vi "New Image (ARGB).vi"(7 "Colour (Default: Black)":T1={"Alpha"=255, "RGB"=0}, 8 "error in (no error)":errorcluster, 11 "Preallocated Image Size (Default: 0,0)":T3) -> (0 "error out":errorcluster, 3 "New ARGB Image":T2)   [LabVIEW 2020, in "g_ar_toolkit.image.lvlib"]
uses:
  g_ar_toolkit.image.lvlib
  g_ar_toolkit.common/Image Size (Integer).ctl
  ARGB Image.ctl
  ARGB Colour.ctl
  3321fa97-f432-4e1e-8db9-a0df79aed21b.vi
  g_ar_toolkit.common/Module Path.vi
  <vilib>/Utility/error.llb/Error Cluster From Error Code.vi
  g_ar_toolkit.common/g_ar_toolkit.common.lvlib
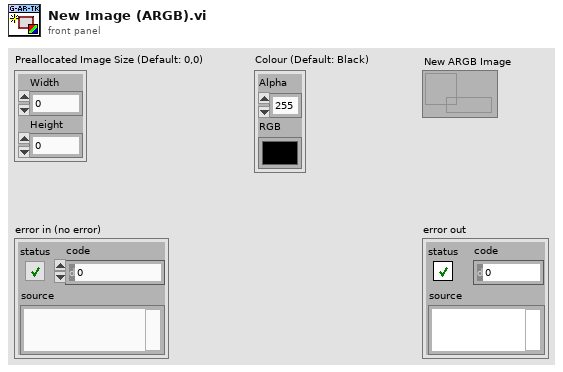
[diagram p1: front panel]
types:
  T1 = typedef "g_ar_toolkit.image.lvlib/ARGB Colour.ctl" = cluster{"Alpha":u8, "RGB":u32}
  T2 = typedef "g_ar_toolkit.image.lvlib/ARGB Image.ctl" = refnum<data-value>
  T3 = typedef "g_ar_toolkit.common.lvlib/Image Size (Integer).ctl" = cluster{"Width":u16, "Height":u16}
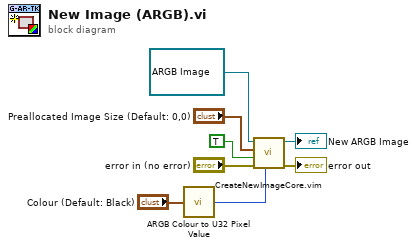
[diagram p0: block diagram]
diagram:
  n1 = call "ARGB Colour to U32 Pixel Value.vi"("ARGB Colour"="Colour (Default: Black)") -> ("U32 Colour"=w1:u32)
  n2 = call "CreateNewImageCore.vim"("Initial Value"=w1, "error in (no error)"="error in (no error)", "Is ARGB"=TRUE, "Preallocated Image Size"="Preallocated Image Size (Default: 0,0)", "Ref Type"=T2 refnum ("EDVR")) -> ("error out"=→"error out":errorcluster, "New Reference"=→"New ARGB Image":T2)  [unwired: 5 in]
